vi "final16_starter.vi"() -> ()   [LabVIEW 2019]
uses:
  <vilib>/Analysis/NI_AALBase.lvlib
  <vilib>/Instr/_visa.llb/VISA Configure Serial Port (Instr).vi
  <vilib>/Utility/file.llb/Write Delimited Spreadsheet (DBL).vi
panel:
  out "Conversion [g]":dbl
  out "Debug array":string[](array[string])
  in  "Stop":bool
  in  "Cycles":dbl min=1.0 step=1.0
  in  "Start operation":bool
  out "String passed to Arduino":string
  in  "Function":u16(ring) items=["Read data ", "Compare different gains", "Execute calibration"]
  out "Received data":string
  in  "Gain":u16(ring) items=["32", "64", "128"]
  out "mean":dbl format="%0.2f"
  out "variance":dbl format="%0.2f"
  out "standard deviation":dbl format="%0.2f"
  in  "Save data path":path
  in  "Arduino COM port":refnum<visa-resource-name>="COM6"
  # "Select all options, then press \"Start operation\" button"
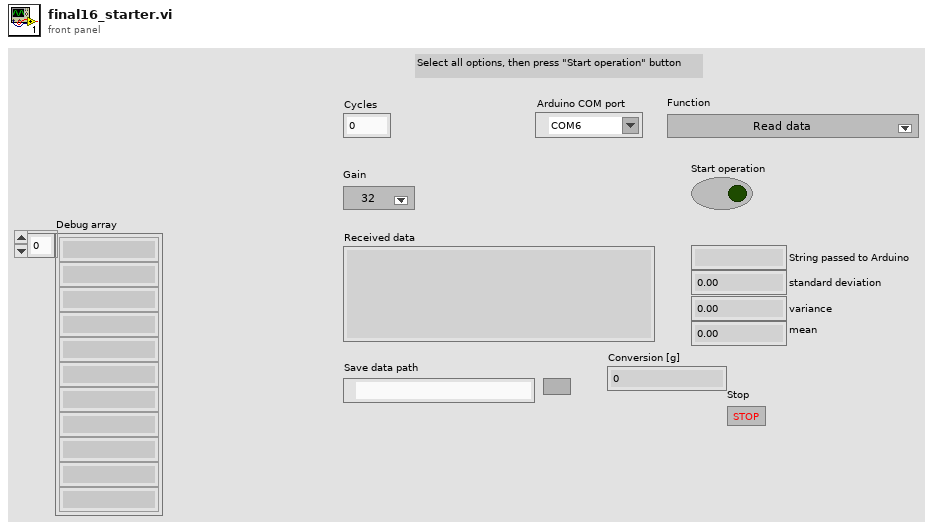
[diagram p1: front panel]
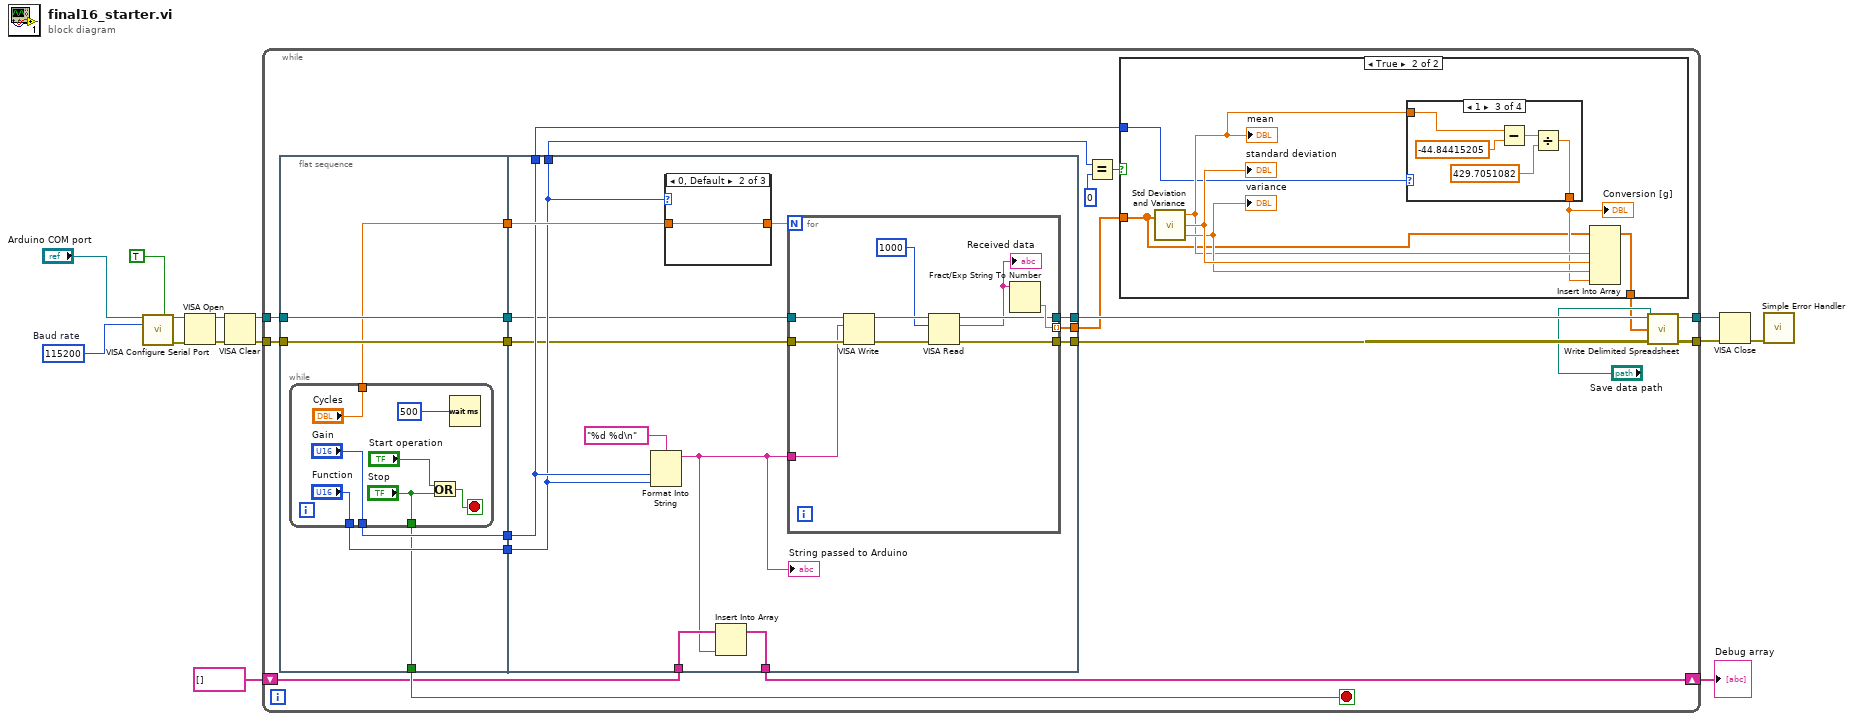
[diagram p0: block diagram]
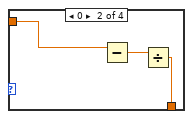
[diagram p4: hidden frame]
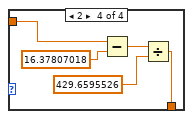
[diagram p5: hidden frame]
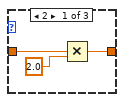
[diagram p6: hidden frame]
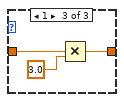
[diagram p7: hidden frame]
diagram:
  w13 = u32 115200  # Baud rate
  n1 = call-poly "VISA Configure Serial Port"("VISA resource name"="Arduino COM port", "Enable Termination\nChar (T)"=TRUE ("Enable Termination\nChar (T)"), "baud rate (9600)"=w13) -> ("VISA resource name out"=w11:refnum<visa-resource-name>, "error out"=w12:errorcluster)  [unwired: 11 in]
  n2 = VISA Open(error in (no error)=w12, VISA resource name=w11) -> (VISA resource name=w8:refnum<visa-resource-name>, error out=w9:errorcluster)  [unwired: 3 in]
  n3 = VISA Clear(VISA resource name=w8, error in (no error)=w9) -> (VISA resource name out=w6:refnum<visa-resource-name>, error out=w7:errorcluster)
  n4 = while {
    tunnel: w7 -> [w34]
    tunnel: w6 -> [w33]
    shift-right: [w27] -> w4
    shift-left: string[] [] -> [w21]
    tunnel: [w25] -> w3
    tunnel: [w22] -> w2
    stop <- w26 stop-if-true
    n5 = flat-sequence {
      tunnel: [w62] -> w32
      tunnel: [w61] -> w31
      tunnel: [w60] -> w30
      tunnel: [w59] -> w29
      tunnel: w34 -> [w61]
      tunnel: w33 -> [w62]
      tunnel: [w58] -> w28
      tunnel: [w57] -> w26
      tunnel: [w82] -> w25
      tunnel: [w81] -> w23
      tunnel: [w80] -> w19
      tunnel: w31 -> [w70]
      tunnel: w32 -> [w71]
      tunnel: w30 -> [w72]
      tunnel: w29 -> [w73]
      tunnel: w28 -> [w77]
      tunnel: [w74] -> w27
      tunnel: w21 -> [w76]
      tunnel: [w73] -> w18
      tunnel: [w72] -> w17
      frame #0 {
        n6 = while {
          tunnel: ["Function"] -> w60
          tunnel: ["Gain"] -> w59
          tunnel: ["Cycles"] -> w58
          tunnel: ["Stop"] -> w57
          stop <- w64 stop-if-true
          n7 = Or(x="Start operation", y="Stop") -> (x .or. y?=w64:bool)
          n8 = Wait (ms)(milliseconds to wait=u32 500) -> ()  [unwired: 1 out]
        }
      }
      frame #1 {
        n9 = Format Into String(format string="%d %d\n", w73, w72) -> (resulting string=w75:string)  [unwired: 2 in, 1 out]
        "String passed to Arduino" <- w75
        n10 = case shown="0, Default" w72 {
          tunnel: w77 -> [w85 w86 w87]
          tunnel: [w83 w86 w88] -> w78
          frame 2 {
            n11 = Multiply(x=w85, y=2.0) -> (x*y=w83:dbl)
          }
          frame 0, Default {
          }
          frame 1 {
            n12 = Multiply(x=w87, y=3.0) -> (x*y=w88:dbl)
          }
        }
        n13 = Insert Into Array(array=w76, new element=w75) -> (w74:string[])  [unwired: 1 in]
        n14 = for {
          N: w78 -> [_]
          tunnel: [w94] -> w80 mode=indexing
          tunnel: w75 -> [w90]
          tunnel: w71 -> [w96]
          tunnel: [w93] -> w82
          tunnel: w70 -> [w97]
          tunnel: [w95] -> w81
          n15 = VISA Write(VISA resource name=w96, write buffer=w90, error in (no error)=w97) -> (VISA resource name out=w99:refnum<visa-resource-name>, error out=w98:errorcluster)  [unwired: 1 out]
          n16 = VISA Read(VISA resource name=w99, byte count=u32 1000, error in (no error)=w98) -> (VISA resource name out=w93:refnum<visa-resource-name>, read buffer=w92:string, error out=w95:errorcluster)  [unwired: 1 out]
          "Received data" <- w92
          n17 = Fract/Exp String To Number(string=w92) -> (number=w94:dbl)  [unwired: 3 in, 1 out]
        }
      }
    }
    n18 = Equal?(x=w17, y=u16 0) -> (x = y?=w16:bool)
    n19 = case shown="True" w16 {
      tunnel: [w35 w40] -> w20
      tunnel: w19 -> [w35 w36]
      tunnel: w18 -> [_ w37]
      frame False {
      }
      frame True {
        n20 = call <vilib>:"Std Deviation and Variance.vi"("X"=w36) -> ("mean"=w39:dbl, "standard deviation"=w42:dbl, "variance"=w41:dbl)  [unwired: 1 in]
        "standard deviation" <- w42
        "variance" <- w41
        "mean" <- w39
        n21 = case shown="1" w37 {
          tunnel: w39 -> [w43 w46 w47 w52]
          tunnel: [w43 w44 w48 w53] -> w38
          frame Default {
          }
          frame 0 {
            n22 = Subtract(x=w46) -> (x-y=w45:dbl)  [unwired: 1 in]
            n23 = Divide(x=w45) -> (x/y=w44:dbl)  [unwired: 1 in]
          }
          frame 1 {
            n24 = Subtract(x=w47, y=-44.84415205) -> (x-y=w50:dbl)
            n25 = Divide(x=w50, y=429.7051082) -> (x/y=w48:dbl)
          }
          frame 2 {
            n26 = Subtract(x=w52, y=16.37807018) -> (x-y=w55:dbl)
            n27 = Divide(x=w55, y=429.6595526) -> (x/y=w53:dbl)
          }
        }
        "Conversion [g]" <- w38
        n28 = Insert Into Array(array=w36, new element #1=w39, new element #2=w42, new element #3=w41, new element #4=w38) -> (w40:dbl[])  [unwired: 1 in]
      }
    }
    n29 = call-poly <vilib>:"Write Delimited Spreadsheet.vi"("file path (dialog if empty)"="Save data path", "1D data"=w20, "error in (no error)"=w23) -> ("error out"=w22:errorcluster)  [unwired: 11 in, 1 out]
  }
  "Debug array" <- w4
  n30 = VISA Close(VISA resource name=w3, error in (no error)=w2) -> (error out=w1:errorcluster)
  n31 = call <vilib>:"Simple Error Handler.vi"("error in (no error)"=w1) -> ()  [unwired: 4 in, 5 out]
